vi "Create Observer (polymorphic).vi"   [LabVIEW 2011, in "Messenging.lvlib"]
uses:
  Messenging.lvlib
  ObserverSet.lvclass
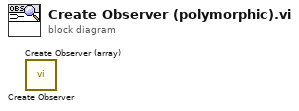
[diagram p0: block diagram]
diagram:
  n1 = call "Create Observer.vi"() -> ()  [unwired: 9 in, 1 out]
  n2 = call "Create Observer (array).vi"() -> ()  [unwired: 9 in, 1 out]
